vi "Start Sync.vi"(8 "error in (no error)":errorcluster, 11 "gRPC Server in":refnum<class "Greeter.lvclass">) -> (0 "error out":errorcluster, 3 "gRPC Server out":refnum<class "Greeter.lvclass">)   [LabVIEW 2019, in "Generated_server.lvlib" / "Greeter.lvclass"]
uses:
  Greeter.lvclass
panel:
  out "error IO":errorcluster
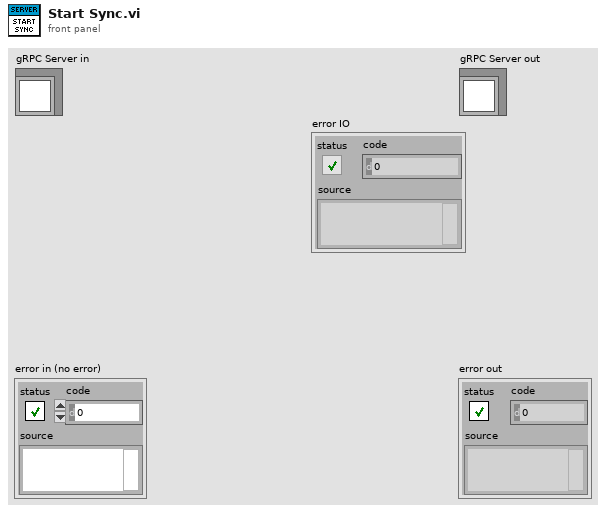
[diagram p1: front panel]
types:
  T1 = typedef "Generated_server.lvlib/Greeter.lvclass/Server Internal UEs.ctl" = cluster{"Greeter SayHello Internal UE":refnum<user-event>, "Greeter SayBye Internal UE":refnum<user-event>}
  T2 = typedef "Generated_server.lvlib/Greeter.lvclass/Server gRPC UEs.ctl" = cluster{"Greeter SayHello gRPC UE":refnum<user-event>, "Greeter SayBye gRPC UE":refnum<user-event>}
  T3 = typedef "grpc-lvsupport-release.lvlib/grpcId.ctl" = u64
  T4 = typedef "Generated_server.lvlib/helloworld_HelloRequest.ctl" = cluster{"name":string}
  T5 = typedef "Generated_server.lvlib/helloworld_ByeRequest.ctl" = cluster{"name":string}
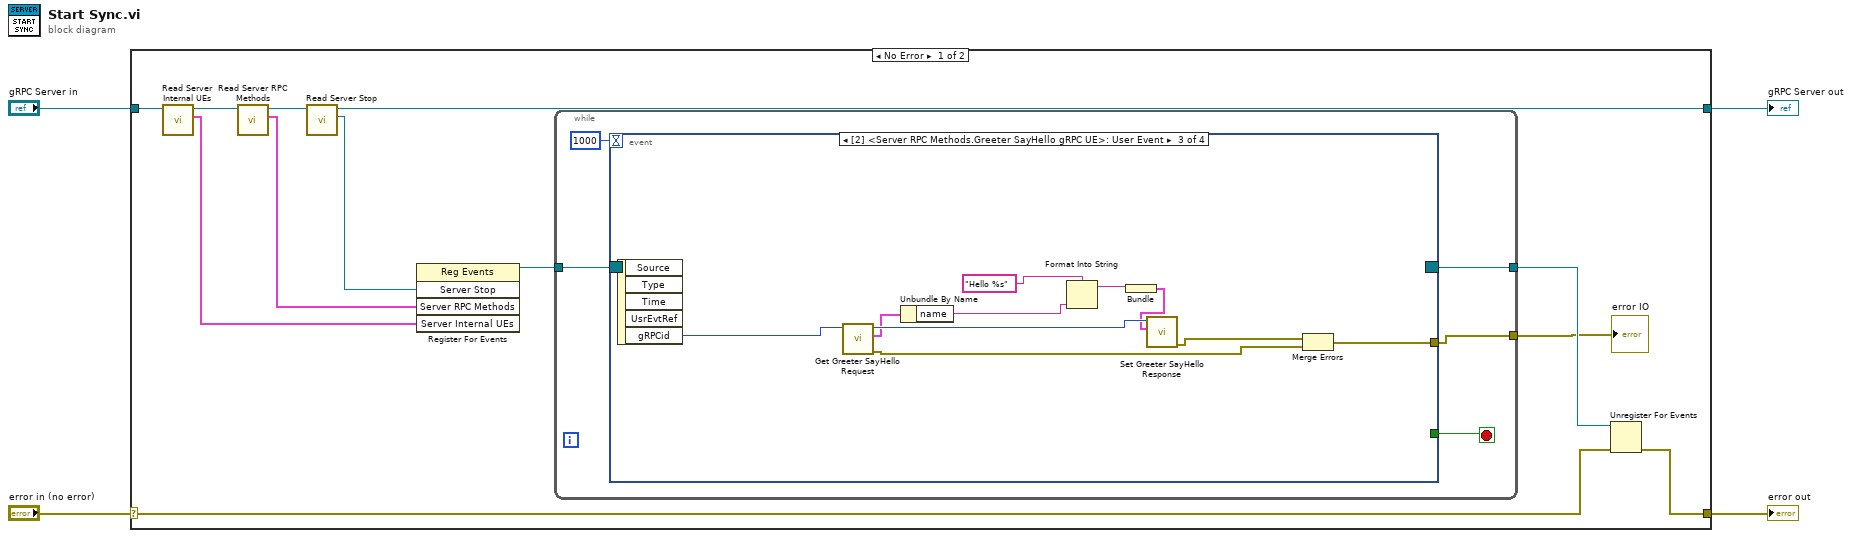
[diagram p0: block diagram]
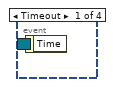
[diagram p2: hidden frame]
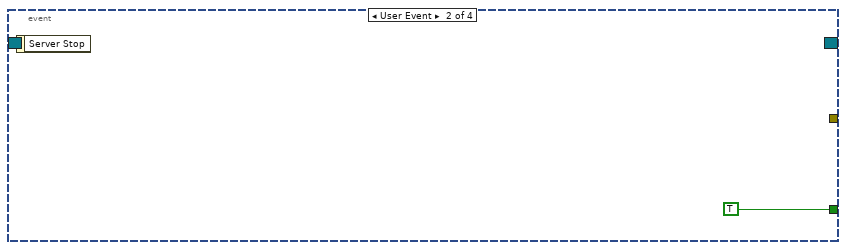
[diagram p3: hidden frame]
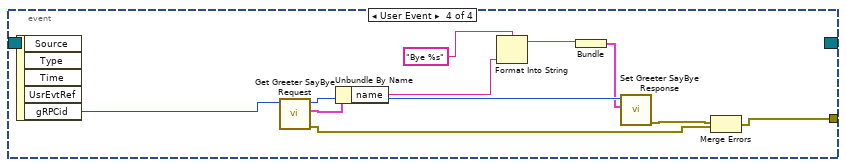
[diagram p4: hidden frame]
diagram:
  n1 = case shown="No Error" "error in (no error)" {
    selector: "error in (no error)" -> [w10 w44]
    tunnel: [w9 w44] -> w3
    tunnel: [w7 w43] -> w1
    tunnel: "gRPC Server in" -> [w16 w43]
    frame No Error {
      n2 = call "Read Server Internal UEs.vi"("SignalGeneratorService in"=w16) -> ("Server Internal UEs"=w14:T1, "SignalGeneratorService out"=w15:refnum<class "Greeter.lvclass">)  [unwired: 8 in, 1 out]
      n3 = call "Read Server RPC Methods.vi"("SignalGeneratorService in"=w15) -> ("Server RPC Methods"=w8:T2, "SignalGeneratorService out"=w13:refnum<class "Greeter.lvclass">)  [unwired: 8 in, 1 out]
      n4 = call-dynamic "Read Server Stop.vi"("iService in"=w13) -> ("Server Stop"=w6:refnum<user-event>, "iService out"=w7:refnum<class "Greeter.lvclass">)  [unwired: 8 in, 1 out]
      n5 = register-events(w6, w8, w14) -> (reference out=w12:refnum<event-registration>)  [unwired: 2 in, 1 out]
      n6 = while {
        tunnel: w12 -> [w21]
        tunnel: [w19] -> w11
        tunnel: [w17] -> w5
        stop <- w20 stop-if-true
        n7 = event "RPC Methods Event Structure" shown="[2] <Server RPC Methods.Greeter SayHello gRPC UE>: User Event" {
          selector: w21 -> [_ _ _ _]
          dyn-events: [_ _ _ _] -> w19
          timeout: 1000 -> [_ _ _ _]
          tunnel: [_ TRUE _ _] -> w20
          tunnel: [_ _ w24 w34] -> w17
          event Timeout {
            n8 = event-data() -> ()  [unwired: 1 in, 1 out]
          }
          event User Event {
            n9 = event-data() -> ()  [unwired: 1 in, 1 out]
          }
          event User Event {
            n10 = event-data() -> ("gRPCid"=w32:T3)  [unwired: 1 in, 4 out]
            n11 = call "Get Greeter SayHello Request.vi"("gRPCid in"=w32) -> ("error out"=w26:errorcluster, "Message Data"=w30:T4, "gRPCid out"=w31:T3)  [unwired: 8 in]
            n12 = Unbundle By Name(w30) -> ("name"=w29:string)
            n13 = Format Into String(format string="Hello %s", w29) -> (resulting string=w28:string)  [unwired: 2 in, 1 out]
            n14 = Bundle(w28) -> (w27:cluster{string})  [unwired: 1 in]
            n15 = call "Set Greeter SayHello Response.vi"("Message Data"=w27, "gRPCid in"=w31) -> ("error out"=w25:errorcluster)  [unwired: 9 in]
            n16 = Merge Errors(w25, w26) -> (w24:errorcluster)
          }
          event User Event {
            n17 = event-data() -> ("gRPCid"=w42:T3)  [unwired: 1 in, 4 out]
            n18 = call "Get Greeter SayBye Request.vi"("gRPCid in"=w42) -> ("error out"=w36:errorcluster, "Message Data"=w40:T5, "gRPCid out"=w41:T3)  [unwired: 8 in]
            n19 = Unbundle By Name(w40) -> ("name"=w39:string)
            n20 = Format Into String(format string="Bye %s", w39) -> (resulting string=w38:string)  [unwired: 2 in, 1 out]
            n21 = Bundle(w38) -> (w37:cluster{string})  [unwired: 1 in]
            n22 = call "Set Greeter SayBye Response.vi"("Message Data"=w37, "gRPCid in"=w41) -> ("error out"=w35:errorcluster)  [unwired: 9 in]
            n23 = Merge Errors(w35, w36) -> (w34:errorcluster)
          }
        }
      }
      "error IO" <- w5
      n24 = Unregister For Events(event registration refnum=w11, error in=w10) -> (error out=w9:errorcluster)
    }
    frame Error {
    }
  }
  "error out" <- w3
  "gRPC Server out" <- w1
